vi "GetLVSupportBuildSpecPath.vi"(11 "base path":path) -> (3 "build spec path":path)   [LabVIEW 2019]
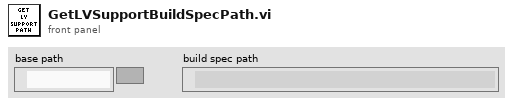
[diagram p1: front panel]
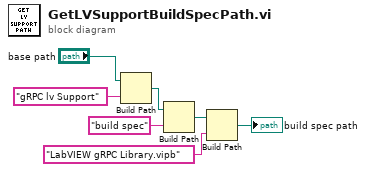
[diagram p0: block diagram]
diagram:
  n1 = Build Path(base path="base path", name or relative path="gRPC lv Support") -> (appended path=w3:path)
  n2 = Build Path(base path=w3, name or relative path="build spec") -> (appended path=w6:path)
  n3 = Build Path(base path=w6, name or relative path="LabVIEW gRPC Library.vipb") -> (appended path=→"build spec path":path)
